vi "Create Log File.vi"(11 "HAL Config Data":T1) -> (1 "String":string, 2 "Byte Stream File out":refnum<file>, 3 "Seconds":dbl)   [LabVIEW 2014]
uses:
  TypeDefs/HAL Config Data.ctl
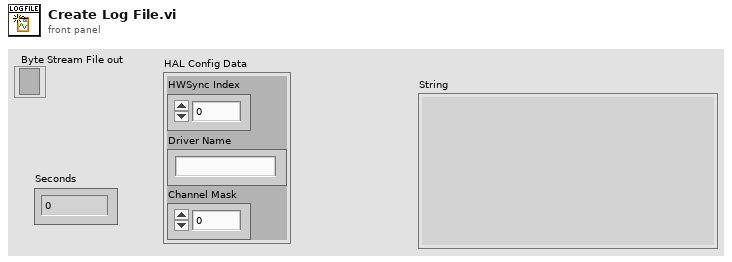
[diagram p1: front panel]
types:
  T1 = typedef "HAL Config Data.ctl" = cluster{"HWSync Index":u32, "Driver Name":string, "Channel Mask":u64}
  T2 = enum16{"open", "replace", "create", "open or create", "replace or create", "replace or create with confirmation"}
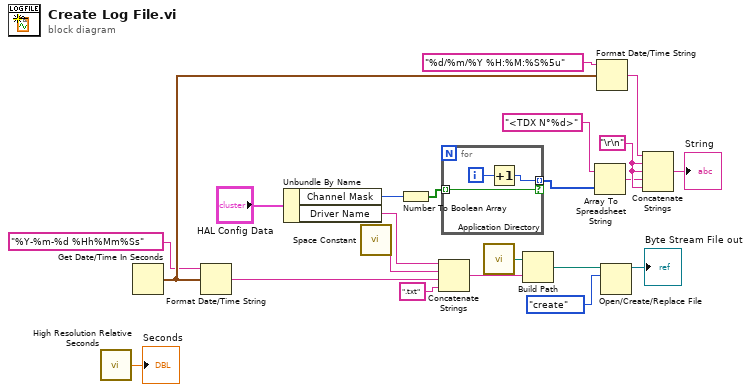
[diagram p0: block diagram]
diagram:
  w6 = "\r\n"
  n1 = call <vilib>:"High Resolution Relative Seconds.vi"() -> ("relative seconds"=→"Seconds":dbl)
  n2 = Get Date/Time In Seconds() -> (seconds since 1Jan1904=w22:timestamp)
  n3 = Format Date/Time String(time format string (%c)="%Y-%m-%d %Hh%Mm%Ss" ("string"), seconds (now)=w22) -> (date/time string=w19:string)  [unwired: 1 in]
  n4 = Unbundle By Name("HAL Config Data") -> ("Channel Mask"=w3:u64, "Driver Name"=w4:string)
  n5 = call <vilib>:"Space Constant.vi"() -> ("String"=w14:string)
  n6 = Number To Boolean Array(number=w3) -> (Boolean array=w2:bool[])
  n7 = Concatenate Strings(w4, w14, w19, ".txt" ("string")) -> (w17:string)
  n8 = for {
    tunnel: w2 -> [w25] mode=indexing
    tunnel: [w23] -> w1 mode=indexing if=w25
    i -> [w24]
    n9 = Increment(x=w24) -> (x+1=w23:i32)
  }
  n10 = call <vilib>:"Application Directory.vi"() -> ("Application Directory"=w11:path)
  n11 = Build Path(base path=w11, name or relative path=w17) -> (appended path=w12:path)
  n12 = Array To Spreadsheet String(array=w1, 3:"<TDX N°%d>" ("format string")) -> (spreadsheet string=w5:string)  [unwired: 1 in]
  n13 = Format Date/Time String(time format string (%c)="%d/%m/%Y %H:%M:%S%5u" ("string"), seconds (now)=w22) -> (date/time string=w9:string)  [unwired: 1 in]
  n14 = Open/Create/Replace File(file path (use dialog)=w12, operation (0:open)=T2."create") -> (refnum out=→"Byte Stream File out":refnum<file>)  [unwired: 4 in, 2 out]
  n15 = Concatenate Strings(w9, w6, w6, w5, w6) -> (→"String":string)
